vi "IMAQ FPGA Data Valid Bool Array to Int x16.vi"(11 "DV In":bool[](array[boolean])=[FALSE, FALSE, FALSE, FALSE, FALSE, FALSE, FALSE, FALSE, FALSE, FALSE, FALSE, FALSE, FALSE, FALSE, FALSE, FALSE]) -> (3 "DV Out":u8)   [LabVIEW 2020, in "NI_VDM_FPGA_Basics.lvlib"]
uses:
  <vilib>/visionFPGA/NI_VDM_FPGA_Basics.lvlib
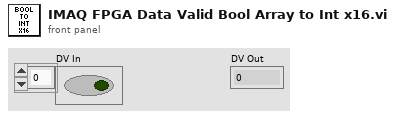
[diagram p1: front panel]
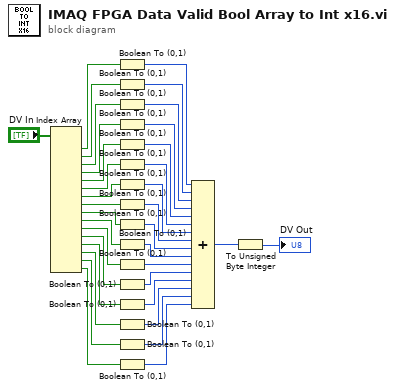
[diagram p0: block diagram]
diagram:
  n1 = Index Array(array="DV In") -> (element #1=w34:bool, element #2=w33:bool, element #3=w32:bool, element #4=w31:bool, element #5=w30:bool, element #6=w29:bool, element #7=w28:bool, element #8=w27:bool, element #9=w17:bool, element #10=w16:bool, element #11=w15:bool, element #12=w14:bool, element #13=w13:bool, element #14=w12:bool, element #15=w11:bool, element #16=w10:bool)  [unwired: 16 in]
  n2 = Boolean To (0,1)(Boolean=w34) -> (0, 1=w26:i16)
  n3 = Boolean To (0,1)(Boolean=w33) -> (0, 1=w25:i16)
  n4 = Boolean To (0,1)(Boolean=w32) -> (0, 1=w24:i16)
  n5 = Boolean To (0,1)(Boolean=w31) -> (0, 1=w23:i16)
  n6 = Boolean To (0,1)(Boolean=w30) -> (0, 1=w22:i16)
  n7 = Boolean To (0,1)(Boolean=w29) -> (0, 1=w21:i16)
  n8 = Boolean To (0,1)(Boolean=w28) -> (0, 1=w20:i16)
  n9 = Boolean To (0,1)(Boolean=w27) -> (0, 1=w19:i16)
  n10 = Boolean To (0,1)(Boolean=w17) -> (0, 1=w9:i16)
  n11 = Boolean To (0,1)(Boolean=w16) -> (0, 1=w8:i16)
  n12 = Boolean To (0,1)(Boolean=w15) -> (0, 1=w7:i16)
  n13 = Boolean To (0,1)(Boolean=w14) -> (0, 1=w6:i16)
  n14 = Boolean To (0,1)(Boolean=w13) -> (0, 1=w5:i16)
  n15 = Boolean To (0,1)(Boolean=w12) -> (0, 1=w4:i16)
  n16 = Boolean To (0,1)(Boolean=w11) -> (0, 1=w3:i16)
  n17 = Boolean To (0,1)(Boolean=w10) -> (0, 1=w2:i16)
  n18 = Compound Arithmetic op=ADD(w26, w25, w24, w23, w22, w21, w20, w19, w9, w8, w7, w6, w5, w4, w3, w2) -> (w18:i16)
  n19 = To Unsigned Byte Integer(number=w18) -> (unsigned 8bit integer=→"DV Out":u8)
